vi "DecisionTree.vi"() -> ()   [LabVIEW 2011]
uses:
  2 Typedefs/setpoints to boat.ctl
  2 Typedefs/sail setpt.ctl
  2 Typedefs/rudder angle.ctl
panel:
  out "Setpoints Out":T1
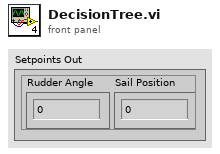
[diagram p1: front panel]
types:
  T1 = typedef "setpoints to boat.ctl" = cluster{"Sail Position":T2, "Rudder Angle":T3}
  T2 = typedef "sail setpt.ctl" = dbl
  T3 = typedef "rudder angle.ctl" = dbl
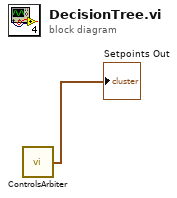
[diagram p0: block diagram]
diagram:
  n1 = call "ControlsArbiter.vi"() -> ("Final Setpoints"=→"Setpoints Out":T1)  [unwired: 15 in]
